vi "Remove SLSC Switch Custom Device.vi"(8 "error in":errorcluster, 11 "slsc switch custom device":T1 format="%.0x") -> (0 "error out":errorcluster)   [LabVIEW 2020, in "SLSC Switch Scripting.lvlib"]
doc: "Removes the SLSC Switch custom device from the owning SLSC chassis. This resets the slot to an empty module."
uses:
  SLSC Switch Scripting.lvlib
  <vilib>/NI VeriStand/Custom Device API/Custom Device Item Ref.ctl
  VeriStand SLSC Scripting API/VeriStand SLSC Scripting.lvlib
  <vilib>/NI VeriStand/Custom Device API/Custom Device API.lvlib
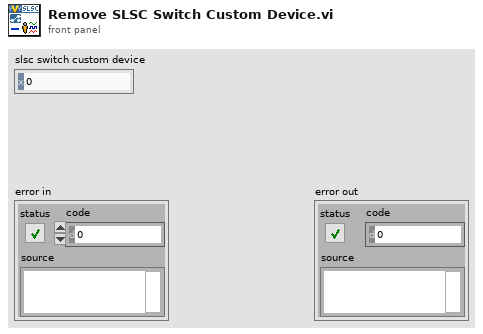
[diagram p1: front panel]
types:
  T1 = typedef "Custom Device API.lvlib/Custom Device Item Ref.ctl" = u64
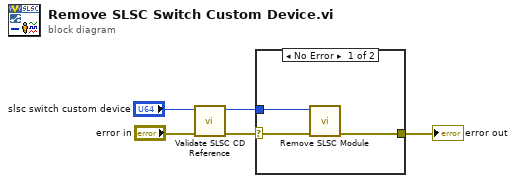
[diagram p0: block diagram]
diagram:
  n1 = call "Validate SLSC CD Reference.vi"("error in"="error in", "slsc switch custom device in"="slsc switch custom device") -> ("error out"=w3:errorcluster, "slsc switch custom device out"=w1:T1)  [unwired: 8 in]
  n2 = case shown="No Error" w3 {
    selector: w3 -> [w6 w9]
    tunnel: [w8 w9] -> w5
    tunnel: w1 -> [w7 _]
    frame No Error {
      n3 = call "Remove SLSC Module.vi"("error in (no error)"=w6, "SLSC Module"=w7) -> ("error out"=w8:errorcluster)  [unwired: 8 in, 1 out]
    }
    frame Error {
    }
  }
  "error out" <- w5
